vi "LVFinal-backup.vi"() -> ()   [LabVIEW 2016]
panel:
  in  "Send Button":bool
  in  "DAC2":dbl
  in  "DAC1":dbl
  out "Angle":dbl
  out "Velocity":dbl
  out "Y":dbl
  out "X":dbl
  in  "stop":bool
  in  "Radius":i16
  in  "Display History":bool
  out "2D Picture":picture
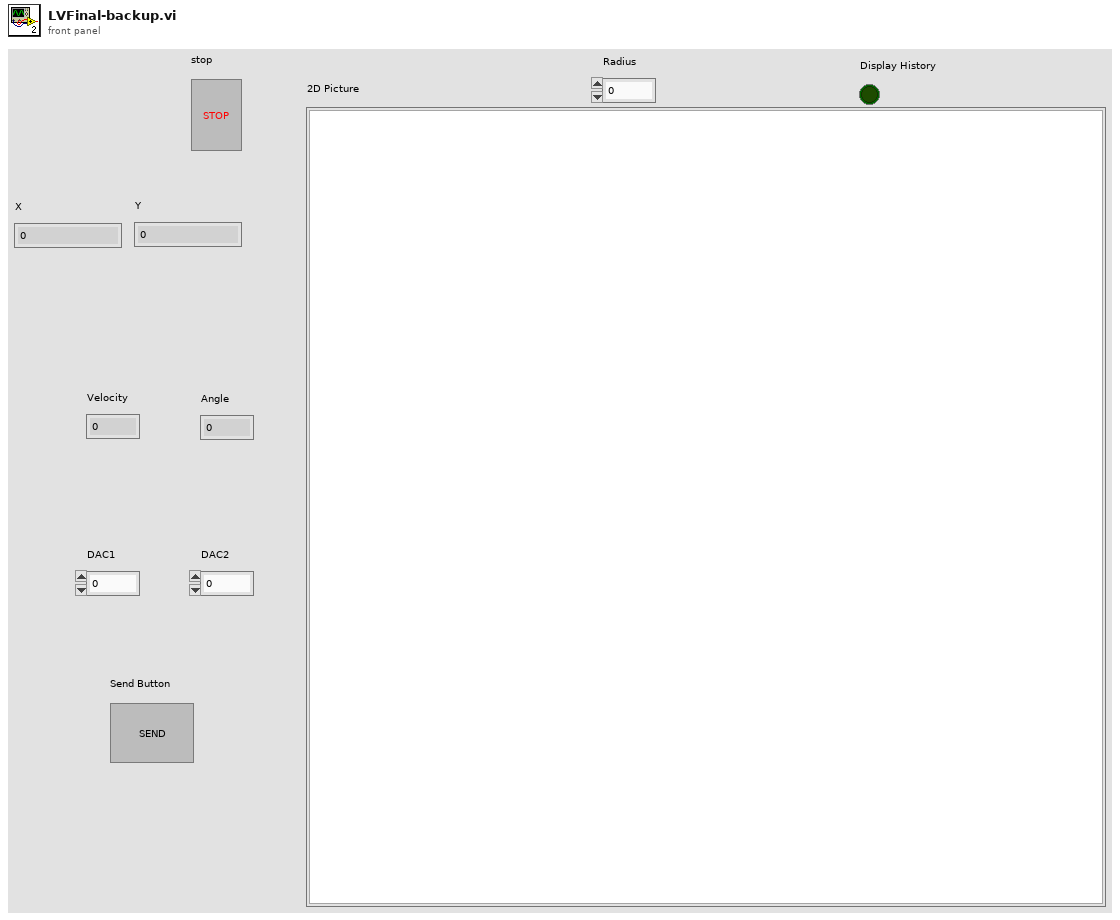
[diagram p1: front panel]
types:
  T1 = cluster{"Width":u16, "Style":enum32{"Solid", "Dash", "Dot", "DashDot", "DashDotDot"}}
  T2 = enum16{"Standard", "Buffered", "CRLF", "Immediate"}
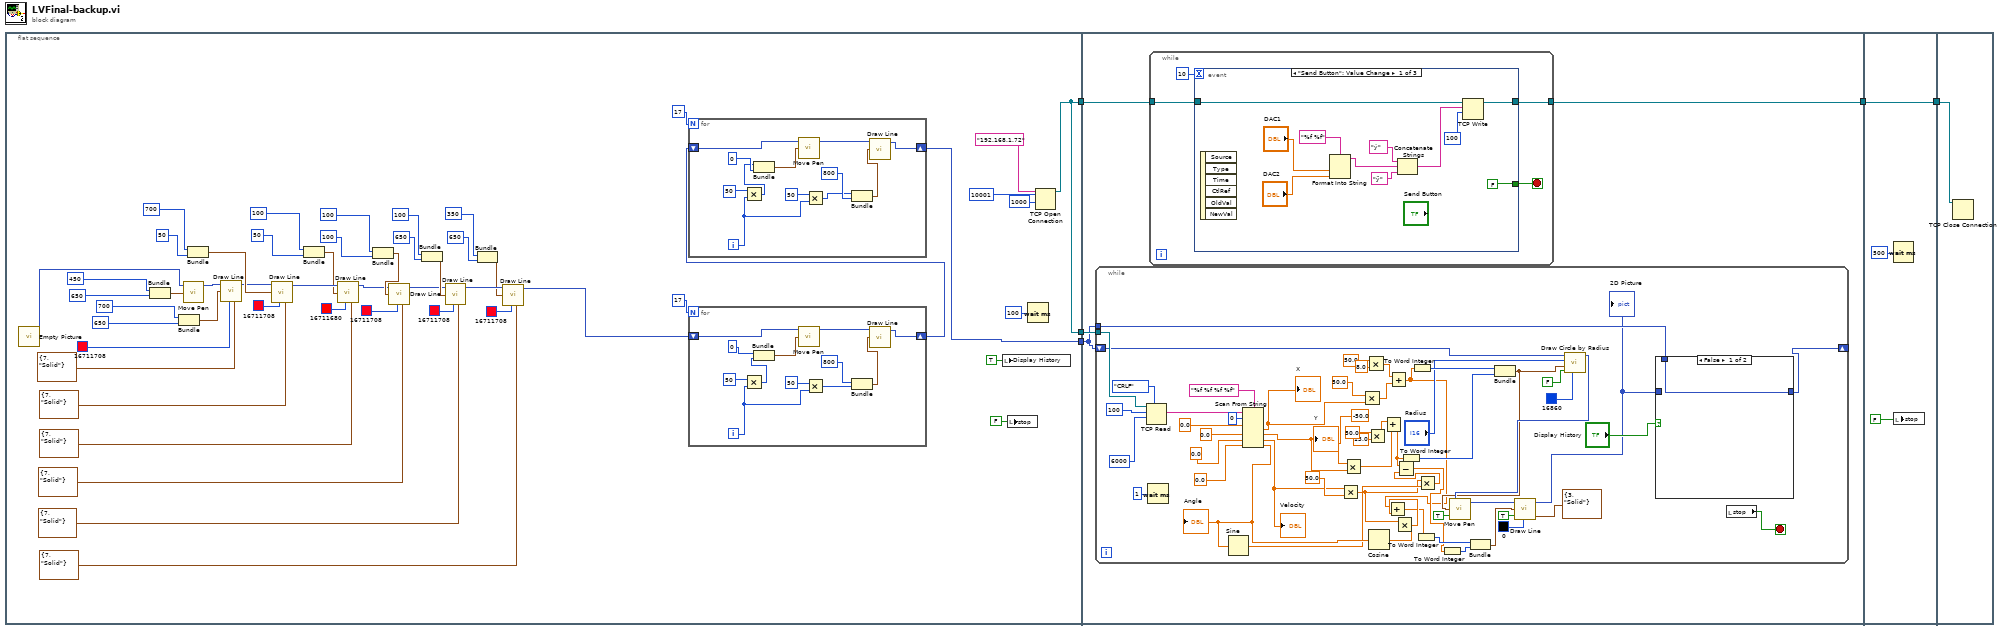
[diagram p0: block diagram]
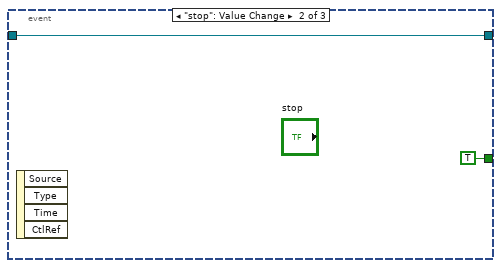
[diagram p3: hidden frame]
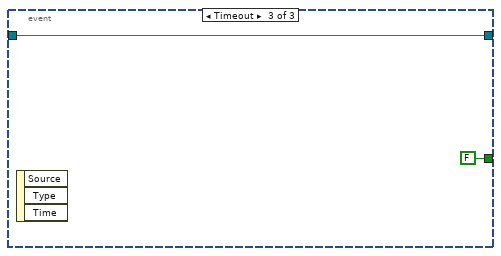
[diagram p4: hidden frame]
diagram:
  n1 = flat-sequence {
    tunnel: [w51] -> w5
    tunnel: [w47] -> w2
    tunnel: [w51] -> w1
    tunnel: w5 -> [w85]
    tunnel: [w84] -> w3
    tunnel: w2 -> [w82]
    tunnel: w1 -> [w83]
    tunnel: [w164] -> w4
    tunnel: w3 -> [w164]
    tunnel: w4 -> [w167]
    frame #0 {
      n2 = call "Empty Picture"() -> ("empty picture"=w39:picture)
      n3 = Bundle(450, 650) -> (w46:cluster{i32, i32})  [unwired: 1 in]
      n4 = Bundle(700, 650) -> (w40:cluster{i32, i32})  [unwired: 1 in]
      n5 = call <vilib>:"Move Pen.vi"("new position"=w46, "picture"=w39) -> ("new picture"=w43:picture)  [unwired: 3 in]
      n6 = Bundle(700, 50) -> (w36:cluster{i32, i32})  [unwired: 1 in]
      n7 = call <vilib>:"Draw Line.vi"("picture"=w43, "end point"=w40, "color(black)"=u32 16711708, "pen"=T1 {"Width"=7, "Style"=enum."Solid"}) -> ("new picture"=w31:picture)  [unwired: 5 in]
      n8 = call <vilib>:"Draw Line.vi"("picture"=w31, "end point"=w36, "color(black)"=u32 16711708, "pen"=T1 {"Width"=7, "Style"=enum."Solid"}) -> ("new picture"=w30:picture)  [unwired: 5 in]
      n9 = Bundle(100, 50) -> (w27:cluster{i32, i32})  [unwired: 1 in]
      n10 = call <vilib>:"Draw Line.vi"("picture"=w30, "end point"=w27, "color(black)"=u32 16711680, "pen"=T1 {"Width"=7, "Style"=enum."Solid"}) -> ("new picture"=w21:picture)  [unwired: 5 in]
      n11 = Bundle(100, 100) -> (w22:cluster{i32, i32})  [unwired: 1 in]
      n12 = call <vilib>:"Draw Line.vi"("picture"=w21, "end point"=w22, "color(black)"=u32 16711708, "pen"=T1 {"Width"=7, "Style"=enum."Solid"}) -> ("new picture"=w17:picture)  [unwired: 5 in]
      n13 = Bundle(100, 650) -> (w18:cluster{i32, i32})  [unwired: 1 in]
      n14 = call <vilib>:"Draw Line.vi"("picture"=w17, "end point"=w18, "color(black)"=u32 16711708, "pen"=T1 {"Width"=7, "Style"=enum."Solid"}) -> ("new picture"=w12:picture)  [unwired: 5 in]
      n15 = Bundle(350, 650) -> (w11:cluster{i32, i32})  [unwired: 1 in]
      n16 = call <vilib>:"Draw Line.vi"("picture"=w12, "end point"=w11, "color(black)"=u32 16711708, "pen"=T1 {"Width"=7, "Style"=enum."Solid"}) -> ("new picture"=w6:picture)  [unwired: 5 in]
      n17 = for {
        N: 17 -> [_]
        shift-right: [w70] -> w48
        shift-left: w6 -> [w72]
        i -> [w71]
        n18 = Multiply(x=50, y=w71) -> (x*y=w74:i32)
        n19 = Bundle(0, w74) -> (w73:cluster{i32, i32})  [unwired: 1 in]
        n20 = call <vilib>:"Move Pen.vi"("new position"=w73, "picture"=w72) -> ("new picture"=w81:picture)  [unwired: 3 in]
        n21 = Multiply(x=50, y=w71) -> (x*y=w79:i32)
        n22 = Bundle(800, w79) -> (w77:cluster{i32, i32})  [unwired: 1 in]
        n23 = call <vilib>:"Draw Line.vi"("picture"=w81, "end point"=w77) -> ("new picture"=w70:picture)  [unwired: 7 in]
      }
      n24 = for {
        N: 17 -> [_]
        shift-right: [w62] -> w47
        shift-left: w48 -> [w64]
        i -> [w63]
        n25 = Multiply(x=50, y=w63) -> (x*y=w60:i32)
        n26 = Bundle(w60, 0) -> (w65:cluster{i32, i32})  [unwired: 1 in]
        n27 = call <vilib>:"Move Pen.vi"("new position"=w65, "picture"=w64) -> ("new picture"=w69:picture)  [unwired: 3 in]
        n28 = Multiply(x=50, y=w63) -> (x*y=w58:i32)
        n29 = Bundle(w58, 800) -> (w67:cluster{i32, i32})  [unwired: 1 in]
        n30 = call <vilib>:"Draw Line.vi"("picture"=w69, "end point"=w67) -> ("new picture"=w62:picture)  [unwired: 7 in]
      }
      n31 = local write "Display History"(TRUE ("Display History")) -> ()
      n32 = local write "stop"(FALSE ("stop")) -> ()
      n33 = Wait (ms)(milliseconds to wait=u32 100) -> ()  [unwired: 1 out]
      n34 = TCP Open Connection(address="192.168.1.72", remote port or service name=u16 10001, timeout ms (60000)=1000) -> (connection ID=w51:refnum<k5>)  [unwired: 2 in, 1 out]
    }
    frame #1 {
      n35 = while {
        shift-right: [w129] -> _
        shift-left: w82 -> [w116]
        tunnel: w83 -> [w128]
        tunnel: w82 -> [w127]
        stop <- w142 stop-if-true
        n36 = TCP Read(connection ID=w128, bytes to read=100, 7:T2."CRLF" ("mode (standard)"), 9:6000 ("timeout ms (25000)")) -> (data out=w137:string)  [unwired: 1 in, 2 out]
        n37 = Wait (ms)(milliseconds to wait=u32 1) -> ()  [unwired: 1 out]
        n38 = Scan From String(format string="%f %f %f %f", input string=w137, initial scan location=u32 0, default 1=0.0 ("default value 1"), default 2=0.0 ("default value 2"), default 3=0.0 ("default value 3"), default 4=0.0 ("default value 4")) -> (output 1=w97:dbl, output 2=w92:dbl, output 3=w107:dbl, output 4=w106:dbl)  [unwired: 1 in, 3 out]
        "X" <- w97
        "Y" <- w92
        "Velocity" <- w107
        "Angle" <- w106
        n39 = Sine(x=w106) -> (sin(x)=w105:dbl)
        n40 = Multiply(x=w107, y=50.0 ("x")) -> (x*y=w102:dbl)
        n41 = Multiply(x=-50.0, y=w92) -> (x*y=w87:dbl)
        n42 = Multiply(x=50.0, y=w97) -> (x*y=w96:dbl)
        n43 = Multiply(x=50.0, y=8.0) -> (x*y=w93:dbl)
        n44 = Multiply(x=50.0, y=13.0) -> (x*y=w89:dbl)
        n45 = Cosine(x=w106) -> (cos(x)=w108:dbl)
        n46 = Add(x=w89, y=w87) -> (x+y=w86:dbl)
        n47 = Add(x=w93, y=w96) -> (x+y=w88:dbl)
        n48 = Multiply(x=w102, y=w108) -> (x*y=w104:dbl)
        n49 = Add(x=w88, y=w104) -> (x+y=w103:dbl)
        n50 = To Word Integer(number=w86) -> (16bit integer=w110:i16)
        n51 = To Word Integer(number=w88) -> (16bit integer=w126:i16)
        n52 = To Word Integer(number=w103) -> (16bit integer=w118:i16)
        n53 = Multiply(x=w102, y=w105) -> (x*y=w101:dbl)
        n54 = Subtract(x=w86, y=w101) -> (x-y=w100:dbl)
        n55 = To Word Integer(number=w100) -> (16bit integer=w109:i16)
        n56 = Bundle(w118, w109) -> (w111:cluster{i16, i16})  [unwired: 1 in]
        n57 = Bundle(w126, w110) -> (w112:cluster{i16, i16})  [unwired: 1 in]
        n58 = call <vilib>:"Draw Circle by Radius.vi"("color(black)"=u32 16860, "fill?(F)"=FALSE, "pixel center"=w112, "radius"="Radius", "picture"=w116) -> ("new picture"=w115:picture)  [unwired: 6 in]
        n59 = call <vilib>:"Move Pen.vi"("absolute coordinates?(T)"=TRUE, "new position"=w112, "picture"=w115) -> ("new picture"=w114:picture)  [unwired: 2 in]
        n60 = call <vilib>:"Draw Line.vi"("picture"=w114, "end point"=w111, "absolute coordinates?(T)"=TRUE, "color(black)"=u32 0, "pen"=T1 {"Width"=3, "Style"=enum."Solid"}) -> ("new picture"=w113:picture)  [unwired: 4 in]
        "2D Picture" <- w113
        n61 = case shown="False" "Display History" {
          tunnel: w113 -> [_ w144]
          tunnel: [w143 w144] -> w129
          tunnel: w127 -> [w143 _]
          frame False {
          }
          frame True {
          }
        }
        n62 = local read "stop"() -> (w142:bool)
      }
      n63 = while {
        tunnel: w85 -> [w147]
        tunnel: [w146] -> w84
        stop <- w148 stop-if-true
        n64 = event shown="[0] \"Send Button\": Value Change" {
          selector: _ -> [_ _ _]
          dyn-events: _ -> [_ _ _]
          timeout: 10 -> [_ _ _]
          tunnel: [FALSE TRUE FALSE] -> w148
          tunnel: w147 -> [w150 w160 w163]
          tunnel: [w149 w160 w163] -> w146
          event "Send Button": Value Change {
            n65 = event-data() -> ()  [unwired: 1 in, 6 out]
            n66 = Format Into String(format string="%f %f", "DAC1", "DAC2") -> (resulting string=w157:string)  [unwired: 2 in, 1 out]
            n67 = Concatenate Strings("ý" ("string"), w157, "ÿ" ("string")) -> (w152:string)
            n68 = TCP Write(connection ID=w150, data in=w152, 9:100 ("timeout ms (25000)")) -> (connection ID out=w149:refnum<k5>)  [unwired: 1 in, 2 out]
          }
          event "stop": Value Change {
            n69 = event-data() -> ()  [unwired: 1 in, 4 out]
          }
          event Timeout {
            n70 = event-data() -> ()  [unwired: 1 in, 3 out]
          }
        }
      }
    }
    frame #2 {
      n71 = Wait (ms)(milliseconds to wait=u32 500) -> ()  [unwired: 1 out]
      n72 = local write "stop"(FALSE) -> ()
    }
    frame #3 {
      n73 = TCP Close Connection(connection ID=w167) -> ()  [unwired: 2 in, 2 out]
    }
  }
